vi "Calc_Rayleigh.vi"(1 "Wavelength":dbl[](array[numeric])) -> (21 "Rayleigh He":dbl[](array[numeric]), 23 "Rayleigh Ambient":dbl[](array[numeric]))   [LabVIEW 2025]
panel:
  out "Rayleigh Zero":dbl[](array[numeric])
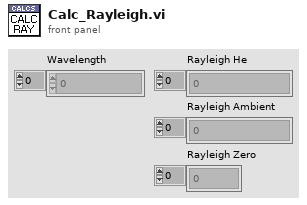
[diagram p1: front panel]
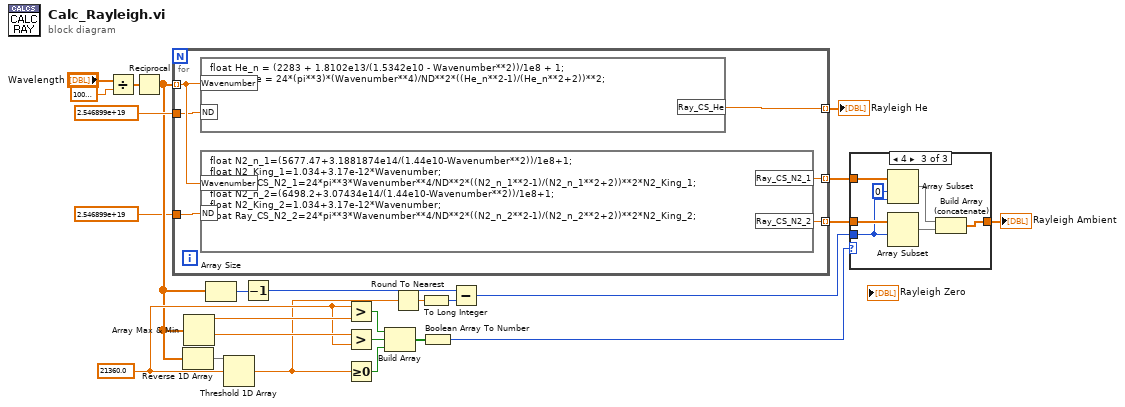
[diagram p0: block diagram]
diagram:
  w18 = 21360.0 ("element")
  n1 = Divide(x="Wavelength", y=10000000.0) -> (x/y=w23:dbl[])
  n2 = Reciprocal(x=w23) -> (1/x=w8:dbl[])
  n3 = for {
    tunnel: w8 -> [w30] mode=indexing
    tunnel: 2.546899e+19 ("ND") -> [w29]
    tunnel: [w31] -> w21 mode=indexing
    tunnel: [w28] -> w11 mode=indexing
    tunnel: [w27] -> w12 mode=indexing
    tunnel: 2.546899e+19 ("ND") -> [w26]
    n4 = formula code="float He_n = (2283 + 1.8102e13/(1.5342e10 - Wavenumber**2))/1e8 + 1;\nRay_CS_He = 24*(pi**3)*(Wavenumber**4)/ND**2*((He_n**2-1)/(He_n**2+2))**2;"("Wavenumber"=w30, "ND"=w29) -> ("Ray_CS_He"=w31:dbl)
    n5 = formula code="float N2_n_1=(5677.47+3.1881874e14/(1.44e10-Wavenumber**2))/1e8+1;\nfloat N2_King_1=1.034+3.17e-12*Wavenumber;\nfloat Ray_CS_N2_1=24*pi**3*Wavenumber**4/ND**2*((N2_n_1**2-1)/(N2_n_1**2+2))**2*N2_King_1;\nfloat N2_n_2=(6498.2+3.07434e14/(1.44e10-Wavenumber**2))/1e8+1;\nfloat N2_King_2=1.034+3.17e-12*Wavenumber;\nfloat Ray_CS_N2_2=24*pi**3*Wavenumber**4/ND**2*((N2_n_2**2-1)/(N2_n_2**2+2))**2*N2_King_2;"("Wavenumber"=w30, "ND"=w26) -> ("Ray_CS_N2_1"=w28:dbl, "Ray_CS_N2_2"=w27:dbl)
  }
  "Rayleigh He" <- w21
  n6 = Reverse 1D Array(array=w8) -> (reversed array=w9:dbl[])
  n7 = Array Max & Min(array=w8) -> (max value=w20:dbl, min value=w19:dbl)  [unwired: 2 out]
  n8 = Array Size(array=w8) -> (size(s)=w4:i32)
  n9 = Threshold 1D Array(2:w18, 3:w9) -> (0:w7:dbl)  [unwired: 1 in]
  n10 = Decrement(x=w4) -> (x-1=w3:i32)
  n11 = Greater?(x=w18, y=w20) -> (0:w17:bool)
  n12 = Greater?(x=w19, y=w18) -> (0:w16:bool)
  n13 = Greater Or Equal To 0?(x=w7) -> (x >= 0?=w15:bool)
  n14 = Build Array(w17, w16, w15) -> (w14:bool[])
  n15 = Round To Nearest(number=w7) -> (nearest integer value=w10:dbl)
  n16 = To Long Integer(number=w10) -> (32bit integer=w5:i32)
  n17 = Boolean Array To Number(Boolean array=w14) -> (number=w13:u32)
  n18 = Subtract(x=w3, y=w5) -> (x-y=w6:i32)
  n19 = case shown="4" w13 {
    tunnel: w12 -> [w32 _ w38]
    tunnel: w11 -> [_ w33 w39]
    tunnel: [w32 w33 w35] -> w2
    tunnel: w6 -> [_ _ w34]
    frame 1, Default {
    }
    frame 2 {
    }
    frame 4 {
      n20 = Array Subset(array=w39, index=0, length=w34) -> (w37:dbl[])
      n21 = Array Subset(array=w38, index=w34) -> (w36:dbl[])  [unwired: 1 in]
      n22 = Build Array (concatenate)(w37, w36) -> (w35:dbl[])
    }
  }
  "Rayleigh Ambient" <- w2
